vi "Kursovaya 3.vi"() -> ()   [LabVIEW 2013]
uses:
  <vilib>/measure/mascope.llb/Transition Measurements 1 chan.vi
  <vilib>/measure/mascope.llb/Pulse Measurements 1 chan.vi
  <vilib>/measure/NI_MAPro.lvlib
panel:
  in  "?":bool
  in  "?":bool
  out "макс значение":dbl[](array[numeric])
  out "Длительность импульса":dbl[](array[numeric])
  out "Время подъема":dbl[](array[numeric])
  in  "?":bool
  in  "?":bool
  out "Вывод ошибки":string
  in  "?":bool
  in  "?":bool
  out "Длительность\nимпульса":dbl format="%.2g"
  out "Время \nподъёма":dbl
  out "?":bool
  out "Наличие \nсигнала":dbl
  out "Мак-ное\nзанчение":dbl
  in  "?":bool
  in  "VISA resource name":refnum<visa-resource-name>
  out "Экран осциллографа":waveform(dbl)(graph)
  in  "Буфер":u32=15000
  in  "Канал (1: Channel 1)":u16(ring)=1 items=["Channel 1"=1, "Channel 2"=2, "Channel 3"=3, "Channel 4"=4]
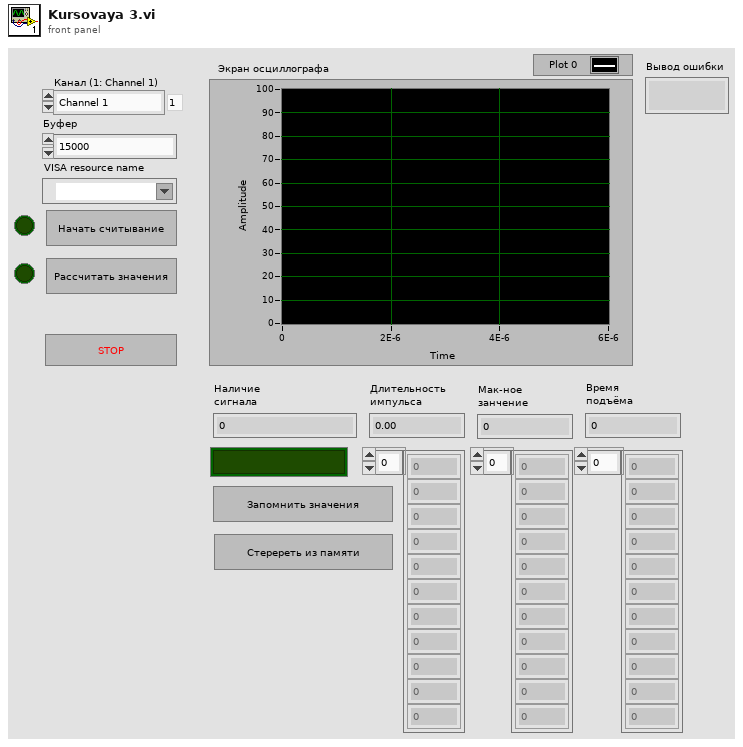
[diagram p1: front panel]
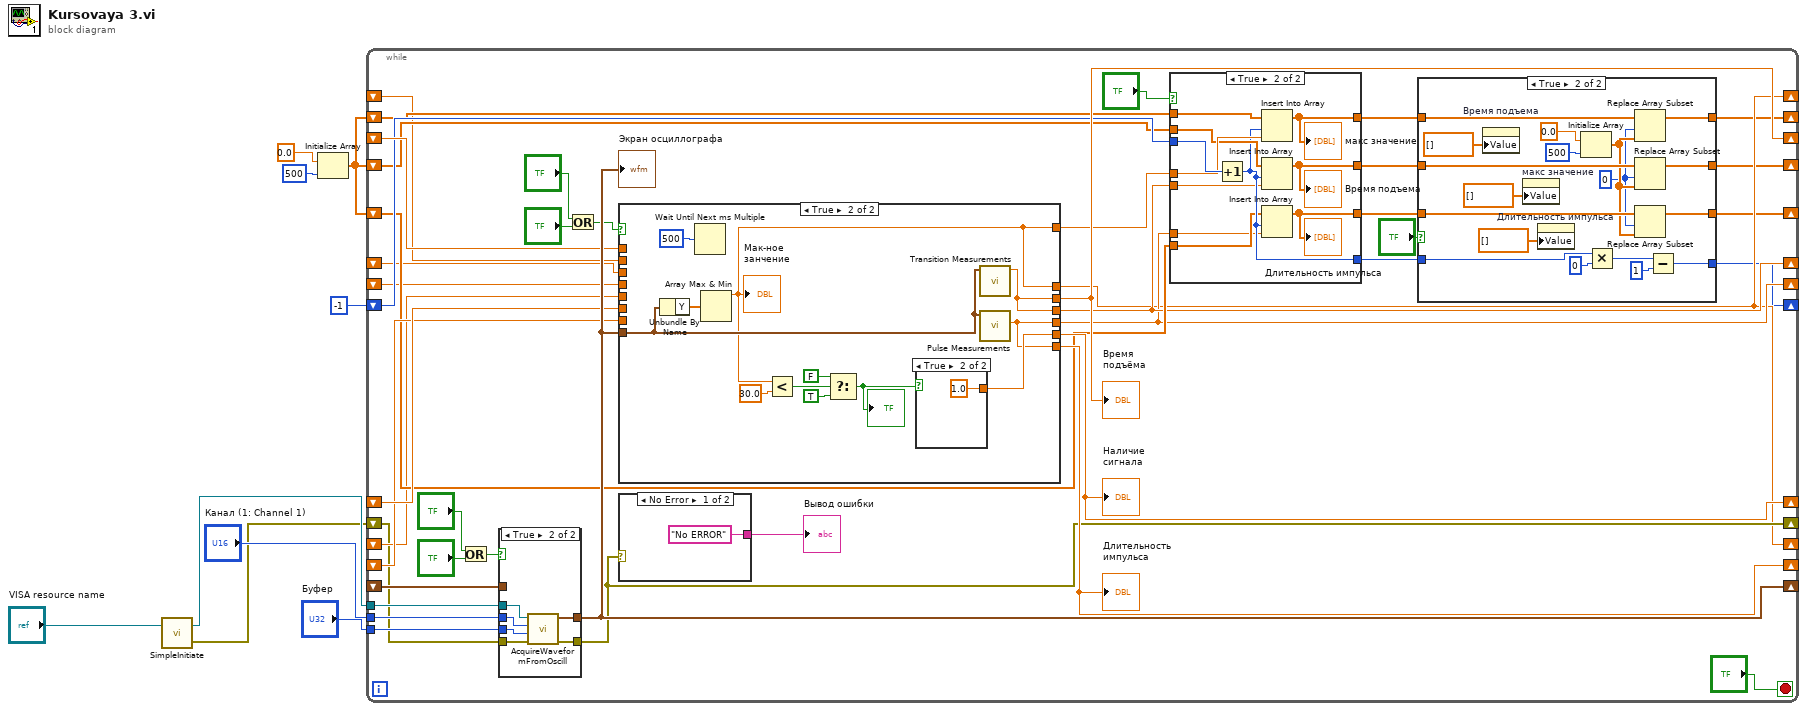
[diagram p0: block diagram]
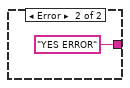
[diagram p4: hidden frame]
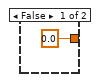
[diagram p6: hidden frame]
diagram:
  n1 = call "SimpleInitiate.vi"("VISA resource name"="VISA resource name") -> ("error out"=w1:errorcluster, "VISA resource name out"=w9:refnum<visa-resource-name>)  [unwired: 1 in]
  n2 = Initialize Array(0.0 ("element"), 500 ("dimension size")) -> (w2:dbl[])
  n3 = while {
    tunnel: w9 -> [w52]
    tunnel: "Канал (1: Channel 1)" -> [w51]
    tunnel: "Буфер" -> [w50]
    shift-right: [w49] -> _
    shift-left: _ -> [w48]
    shift-right: [w41] -> _
    shift-left: w1 -> [w10]
    shift-right: [w47] -> _
    shift-left: _ -> [w46]
    shift-right: [w45] -> _
    shift-left: _ -> [w44]
    shift-right: [w43] -> _
    shift-left: _ -> [w42]
    shift-right: [w17] -> _
    shift-left: -1 -> [w32]
    shift-right: [w19] -> _
    shift-left: w2 -> [w30]
    shift-right: [w14] -> _
    shift-left: w2 -> [w29]
    shift-right: [w13] -> _
    shift-left: w2 -> [w28]
    shift-right: [w22] -> _
    shift-left: _ -> [w27]
    shift-right: [w26] -> _
    shift-left: _ -> [w25]
    shift-right: [w24] -> _
    shift-left: _ -> [w23]
    shift-right: [w22] -> _
    shift-left: _ -> [w21]
    stop <- "?" stop-if-true
    n4 = Or(x="?", y="?") -> (x .or. y?=w37:bool)
    n5 = case shown="True" w37 {
      tunnel: w52 -> [_ w120]
      tunnel: w51 -> [_ w119]
      tunnel: w50 -> [_ w118]
      tunnel: w10 -> [w113 w117]
      tunnel: [w113 w116] -> w41
      tunnel: [w114 w115] -> w49
      tunnel: w48 -> [w114 _]
      frame False {
      }
      frame True {
        n6 = call "AcquireWaveformFromOscill.vi"("error in"=w117, "byte count"=w118, "Channel (1: Channel 1)"=w119, "VISA resource name"=w120) -> ("error out"=w116:errorcluster, "Waveform Graph"=w115:waveform(dbl))  [unwired: 2 out]
      }
    }
    "Экран осциллографа" <- w49
    n7 = Or(x="?", y="?") -> (x .or. y?=w34:bool)
    n8 = case shown="True" w34 {
      tunnel: [w98 w105] -> w47
      tunnel: [w97 w99] -> w45
      tunnel: [w96 w100] -> w43
      tunnel: w49 -> [_ w104]
      tunnel: w46 -> [w98 _]
      tunnel: w44 -> [w97 _]
      tunnel: w42 -> [w96 _]
      tunnel: [w95 w101] -> w31
      tunnel: [w92 w101] -> w22
      tunnel: w27 -> [w95 _]
      tunnel: [w94 w99] -> w26
      tunnel: w25 -> [w94 _]
      tunnel: [w93 w100] -> w24
      tunnel: w23 -> [w93 _]
      tunnel: w21 -> [w92 _]
      frame False {
      }
      frame True {
        n9 = Unbundle By Name(w104) -> ("Y"=w103:dbl[])
        n10 = Wait Until Next ms Multiple(millisecond multiple=u32 500) -> ()  [unwired: 1 out]
        n11 = Array Max & Min(array=w103) -> (max value=w101:dbl)  [unwired: 3 out]
        "Мак-ное\nзанчение" <- w101
        n12 = Less?(x=w101, y=30.0) -> (x < y?=w109:bool)
        n13 = Select(t=FALSE, s=w109, f=TRUE) -> (s? t:f=w106:bool)
        "?" <- w106
        n14 = case shown="True" w106 {
          tunnel: [0.0 ("Numeric") 1.0 ("Numeric")] -> w105
          frame False {
          }
          frame True {
          }
        }
        n15 = call-poly <vilib>:"Transition Measurements.vi"("signal in"=w104) -> ("transition duration"=w99:dbl)  [unwired: 5 in, 5 out]
        n16 = call-poly <vilib>:"Pulse Measurements.vi"("signal in"=w104) -> ("pulse duration"=w100:dbl)  [unwired: 6 in, 4 out]
      }
    }
    "Наличие \nсигнала" <- w47
    "Время \nподъёма" <- w45
    "Длительность\nимпульса" <- w43
    n17 = case shown="No Error" w41 {
      tunnel: ["No ERROR" ("Error") "YES ERROR" ("Error")] -> w40
      frame No Error {
      }
      frame Error {
      }
    }
    "Вывод ошибки" <- w40
    n18 = case shown="True" "?" {
      tunnel: w32 -> [w76 w89]
      tunnel: w31 -> [_ w88]
      tunnel: w30 -> [w78 w87]
      tunnel: [w78 w86] -> w20
      tunnel: w29 -> [w77 w85]
      tunnel: [w77 w84] -> w16
      tunnel: [w76 w83] -> w18
      tunnel: w28 -> [w75 w82]
      tunnel: [w75 w81] -> w15
      tunnel: w26 -> [_ w80]
      tunnel: w24 -> [_ w79]
      frame False {
      }
      frame True {
        n19 = Increment(x=w89) -> (x+1=w83:i32)
        n20 = Insert Into Array(array=w87, index=w83, new element=w88) -> (w86:dbl[])
        "макс значение" <- w86
        n21 = Insert Into Array(array=w85, index=w83, new element=w80) -> (w84:dbl[])
        "Время подъема" <- w84
        n22 = Insert Into Array(array=w82, index=w83, new element=w79) -> (w81:dbl[])
        "Длительность импульса" <- w81
      }
    }
    n23 = case shown="True" "?" {
      tunnel: w20 -> [w56 w74]
      tunnel: [w56 w71] -> w19
      tunnel: w18 -> [w55 w70]
      tunnel: [w55 w66] -> w17
      tunnel: w16 -> [w54 w65]
      tunnel: w15 -> [w53 w64]
      tunnel: [w54 w61] -> w14
      tunnel: [w53 w60] -> w13
      frame False {
      }
      frame True {
        w62 = 0 ("index")
        n24 = property on="Время подъема" class="Arr (strict)"("Value"=dbl[] [] ("Время подъема")) -> ()  [unwired: 2 in, 2 out]
        n25 = property on="макс значение" class="Arr (strict)"("Value"=dbl[] [] ("Время подъема")) -> ()  [unwired: 2 in, 2 out]
        n26 = property on="Длительность импульса" class="Arr (strict)"("Value"=dbl[] [] ("123")) -> ()  [unwired: 2 in, 2 out]
        n27 = Initialize Array(0.0 ("element"), 500 ("dimension size")) -> (w63:dbl[])
        n28 = Multiply(x=w70, y=0) -> (x*y=w68:i32)
        n29 = Replace Array Subset(array=w74, new element=w63, index=w62) -> (w71:dbl[])
        n30 = Replace Array Subset(array=w65, new element=w63, index=w62) -> (w61:dbl[])
        n31 = Replace Array Subset(array=w64, new element=w63, index=w62) -> (w60:dbl[])
        n32 = Subtract(x=w68, y=1) -> (x-y=w66:i32)
      }
    }
  }
